vi "Lookup Part Number Data.vi"(5 "Sequence Context":refnum<k7>) -> (0 "error out":errorcluster, 1 "Cartridge Part Number String":string, 2 "Clent File Path String":string)   [LabVIEW 2010]
uses:
  <vilib>/addons/TestStand/_TSUtility.llb/TestStand - Get Property Value (String).vi
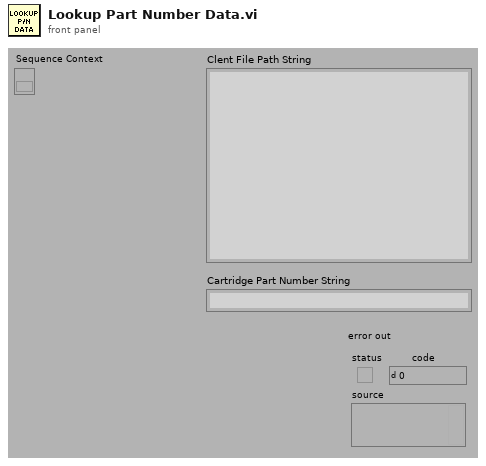
[diagram p1: front panel]
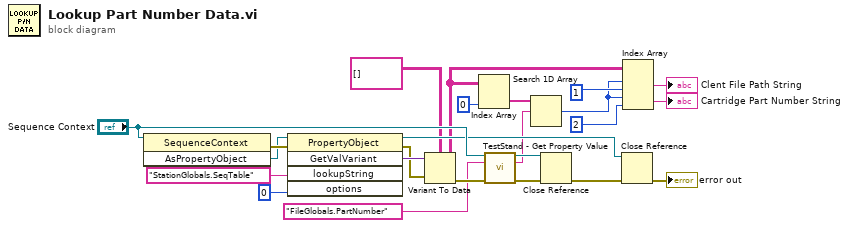
[diagram p0: block diagram]
diagram:
  n1 = invoke class="SequenceContext" method="AsPropertyObject"(reference="Sequence Context") -> (error out=w18:errorcluster, "AsPropertyObject"=w13:refnum<k7>)  [unwired: 2 in, 1 out]
  n2 = invoke class="PropertyObject" method="GetValVariant"(reference=w13, error in=w18, "lookupString"="StationGlobals.SeqTable" ("Lookup String"), "options"=0) -> (reference out=w7:refnum<k7>, error out=w19:errorcluster, "GetValVariant"=w21:variant)  [unwired: 1 in, 2 out]
  n3 = Variant To Data(error in=w19, Variant=w21, type=string[][] []) -> (error out=w12:errorcluster, data=w5:string[][])
  n4 = Index Array(array=w5, index (col)=0 ("disabled index (col)")) -> (element=w17:string[])  [unwired: 1 in]
  n5 = call-poly <vilib>:"TestStand - Get Property Value.vi"("Sequence Context In"="Sequence Context", "Lookup String"="FileGlobals.PartNumber", "error in (no error)"=w12) -> ("Sequence Context Out"=w24:refnum<k7>, "Value"=w4:string, "error out"=w9:errorcluster)  [unwired: 10 in]
  n6 = Search 1D Array(1D array=w17, element=w4) -> (index of element=w3:i32)  [unwired: 1 in]
  n7 = Close Reference(reference=w24, error in (no error)=w9) -> (error out=w10:errorcluster)
  n8 = Close Reference(reference=w7, error in (no error)=w10) -> (error out=→"error out":errorcluster)
  n9 = Index Array(array=w5, index (row) #1=w3, index (col) #1=1 ("index (col)"), index (row) #2=w3, index (col) #2=2 ("disabled index (col)")) -> (element #1=→"Clent File Path String":string, element #2=→"Cartridge Part Number String":string)
